vi "UsrProfiles-Update user profiles list.vi"(8 "error in":errorcluster) -> (0 "error out":errorcluster, 3 "reference out":refnum<vi>)   [LabVIEW 2020]
uses:
  Typedefs/Save-Load enum.ctl
  Globals/gl_UsrProfiles globals.vi
  Global Variables/General Globals.vi
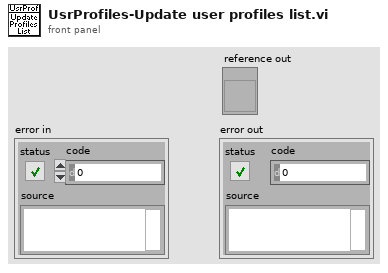
[diagram p1: front panel]
types:
  T1 = typedef "User login window refs.ctl" = cluster{"User profiles window ref":refnum<k9>, "Users listbox":refnum<vi>, "Profiles listbox":refnum<vi>, "Last used":refnum<vi>}
  T2 = typedef "Save-Load enum.ctl" = enum16{"Save to file", "Load from file", "Compare from file", "Save Backup"}
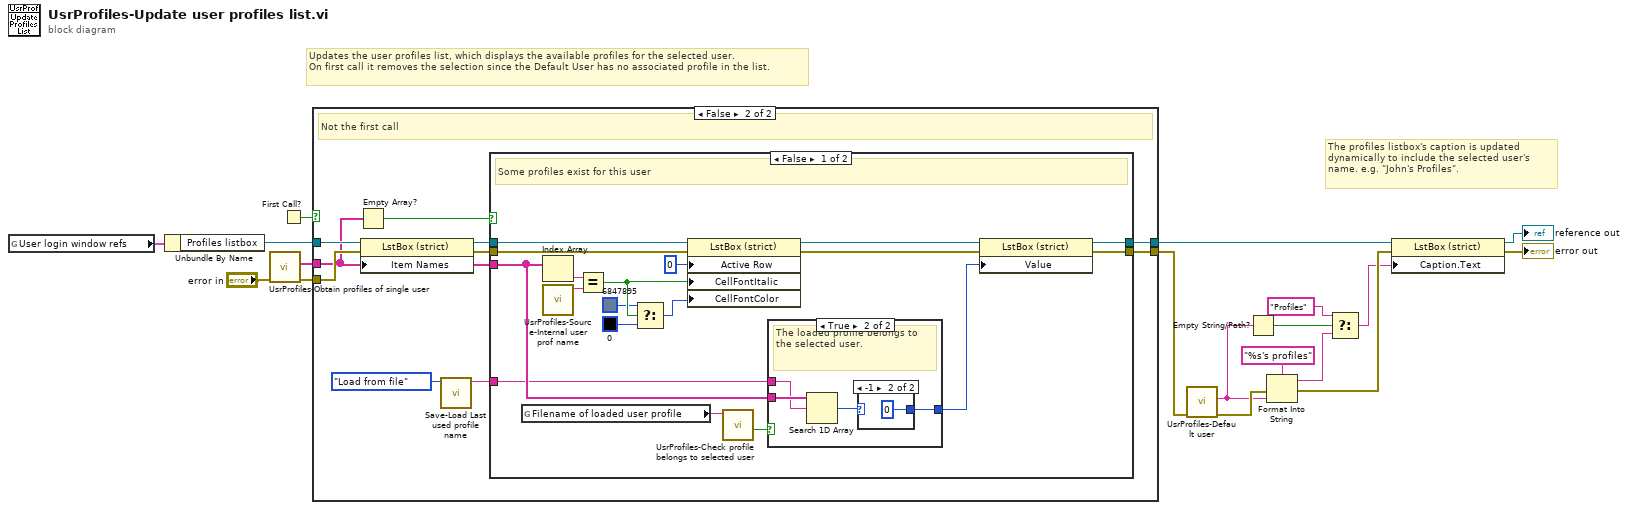
[diagram p0: block diagram]
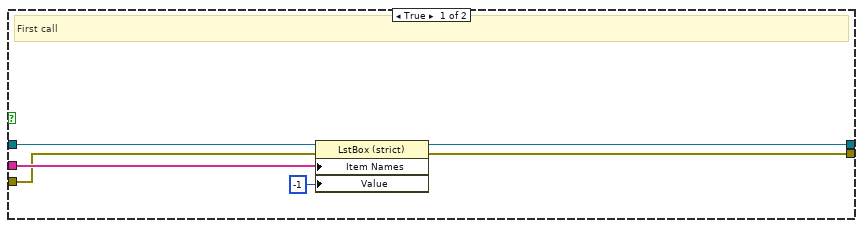
[diagram p2: hidden frame]
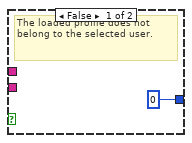
[diagram p3: hidden frame]
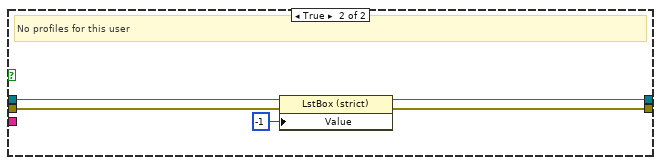
[diagram p5: hidden frame]
diagram:
  # "The profiles listbox's caption is updated dynamically to include the selected user's name. e.g. \"John's Profiles\"."
  # "Updates the user profiles list, which displays the available profiles for the selected user.\nOn first call it removes the selection since the Default User has no associated profile in the list."
  n1 = global read "gl_UsrProfiles globals.vi" "User login window refs"() -> (w15:T1)
  n2 = Unbundle By Name(w15) -> ("Profiles listbox"=w17:refnum<vi>)
  n3 = call "UsrProfiles-Obtain profiles of single user.vi"("error in"="error in") -> ("error out"=w14:errorcluster, "User profile names"=w16:string[])  [unwired: 9 in]
  n4 = First Call?() -> (First Call?: T/F=w18:bool)
  n5 = case shown="False" w18 {
    tunnel: w16 -> [w24 w28]
    tunnel: w17 -> [w23 w34]
    tunnel: [w22 w31] -> w2
    tunnel: w14 -> [w21 w33]
    tunnel: [w19 w26] -> w5
    frame True {
      # "First call"
      n6 = property on="Property Node" class="LstBox (strict)"(reference=w23, error in=w21, "Item Names"=w24, "Value"=-1) -> (reference out=w19:refnum<vi>, error out=w22:errorcluster)
    }
    frame False {
      # "Not the first call"
      n7 = Empty Array?(array=w28) -> (empty?=w29:bool)
      n8 = property on="Property Node" class="LstBox (strict)"(reference=w34, error in=w33, "Item Names"=w28) -> (reference out=w30:refnum<vi>, error out=w32:errorcluster)
      n9 = call "Save-Load Last used profile name.vi"("Function"=Save-Load_enum."Load from file") -> ("Last used profile for selected user"=w27:string)  [unwired: 8 in, 2 out]
      n10 = case shown="False" w29 {
        tunnel: w32 -> [w50 w64]
        tunnel: [w51 w63] -> w31
        tunnel: w30 -> [w52 w62]
        tunnel: w28 -> [w49 _]
        tunnel: w27 -> [w48 _]
        tunnel: [w47 w60] -> w26
        frame False {
          # "Some profiles exist for this user"
          n11 = global read "General Globals.vi" "Filename of loaded user profile"() -> (w37:string)
          n12 = Index Array(array=w49) -> (element=w45:string)  [unwired: 1 in]
          n13 = call "UsrProfiles-Source-Internal user prof name.vi"() -> ("Previous session profile name"=w44:string)  [unwired: 11 in]
          n14 = Equal?(x=w45, y=w44) -> (x = y?=w42:bool)
          n15 = Select(t=u32 6847895 ("Color Box"), s=w42, f=u32 0) -> (s? t:f=w40:u32)
          n16 = property on="Property Node" class="LstBox (strict)"(reference=w52, error in=w50, "Active Row"=0 ("index of element"), "CellFontItalic"=w42, "CellFontColor"=w40) -> (reference out=w39:refnum<vi>, error out=w38:errorcluster)
          n17 = call "UsrProfiles-Check profile belongs to selected user.vi"("Filename of loaded user profile"=w37) -> ("Belongs to selected user"=w36:bool)  [unwired: 10 in]
          n18 = case shown="True" w36 {
            tunnel: [0 w56] -> w35
            tunnel: w49 -> [_ w55]
            tunnel: w48 -> [_ w54]
            frame False {
              # "The loaded profile does not belong to the selected user."
            }
            frame True {
              # "The loaded profile belongs to the selected user."
              n19 = Search 1D Array(1D array=w55, element=w54) -> (index of element=w57:i32)  [unwired: 1 in]
              n20 = case shown="-1" w57 {
                selector: w57 -> [w58 _]
                tunnel: [w58 0] -> w56
                frame Default {
                }
                frame -1 {
                }
              }
            }
          }
          n21 = property on="Property Node" class="LstBox (strict)"(reference=w39, error in=w38, "Value"=w35) -> (reference out=w47:refnum<vi>, error out=w51:errorcluster)
        }
        frame True {
          # "No profiles for this user"
          n22 = property on="Property Node" class="LstBox (strict)"(reference=w62, error in=w64, "Value"=-1) -> (reference out=w60:refnum<vi>, error out=w63:errorcluster)
        }
      }
    }
  }
  n23 = call "UsrProfiles-Default user.vi"("error in (no error)"=w2) -> ("error out"=w4:errorcluster, "Selected user's name"=w3:string)  [unwired: 8 in, 1 out]
  n24 = Empty String/Path?(string/path=w3) -> (empty?=w10:bool)
  n25 = Format Into String(format string="%s's profiles", error in=w4, w3) -> (resulting string=w9:string, error out=w8:errorcluster)  [unwired: 1 in]
  n26 = Select(t="Profiles", s=w10, f=w9) -> (s? t:f=w7:string)
  n27 = property on="Property Node" class="LstBox (strict)"(reference=w5, error in=w8, "Caption.Text"=w7) -> (reference out=→"reference out":refnum<vi>, error out=→"error out":errorcluster)
